vi "Get_MB_Setting.vi"(9 "DeviceName":string, 11 "DBRefNum":i32) -> (0 "Swap":T1, 1 "Mode":enum16{"RTU", "ASCII"}(ring), 2 "Address":string, 3 "DBRefNum Out":i32, 4 "Timeout":i32=1000, 5 "Device Index":u8, 6 "Name":string, 7 "Interval":u32)   [LabVIEW 2020, in "ModBus Serial Master.lvlib"]
uses:
  ModBus Serial Master.lvlib
  DriverCommon/Swap.ctl
  DriverCommon.lvlib
  SQLiteBase.lvlib
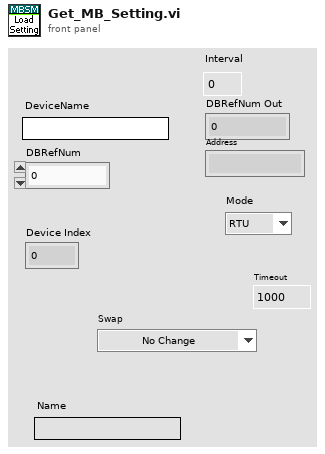
[diagram p1: front panel]
types:
  T1 = typedef "DriverCommon.lvlib/Swap.ctl" = enum16{"No Change", "Swap"}
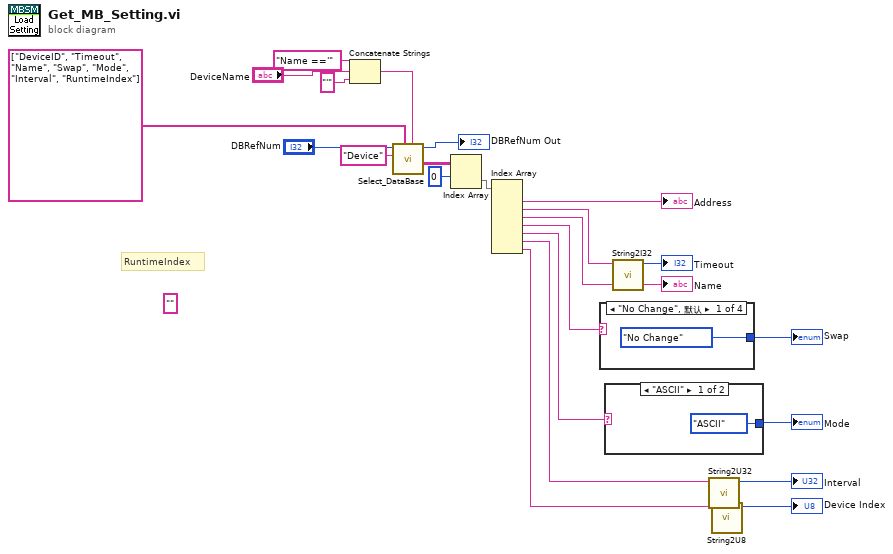
[diagram p0: block diagram]
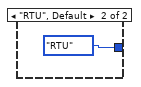
[diagram p2: hidden frame]
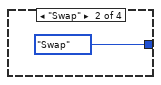
[diagram p3: hidden frame]
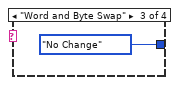
[diagram p4: hidden frame]
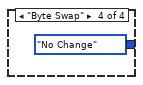
[diagram p5: hidden frame]
diagram:
  (unwired) "" ("Control Name")
  # "RuntimeIndex"
  n1 = Concatenate Strings("Name =='" ("Expression"), "DeviceName", "'" ("string")) -> (w18:string)
  n2 = call "Select_DataBase.vi"("Expression"=w18, "Query Columns"=string[] ["DeviceID", "Timeout", "Name", "Swap", "Mode", "Interval", "RuntimeIndex"], "Table name"="Device", "DB Reference In"="DBRefNum") -> ("Data"=w15:string[][], "DB Reference Out"=→"DBRefNum Out":i32)  [unwired: 5 in, 1 out]
  n3 = Index Array(array=w15, index (row)=0) -> (element=w13:string[])  [unwired: 1 in]
  n4 = Index Array(array=w13) -> (element #1=→"Address":string, element #2=w9:string, element #3=→"Name":string, element #4=w7:string, element #5=w5:string, element #6=w4:string, element #7=w2:string)  [unwired: 7 in]
  n5 = case shown="\"No Change\", 默认" w7 {
    tunnel: [Swap."No Change" ("Swap") Swap."Swap" ("Swap") Swap."No Change" ("Swap") Swap."No Change" ("Swap")] -> w10
    frame "No Change", Default {
    }
    frame "Swap" {
    }
    frame "Word and Byte Swap" {
    }
    frame "Byte Swap" {
    }
  }
  "Swap" <- w10
  n6 = case shown="\"ASCII\"" w5 {
    tunnel: [enum16{"RTU", "ASCII"}."ASCII" ("Mode") enum16{"RTU", "ASCII"}."RTU" ("Mode")] -> w6
    frame "ASCII" {
    }
    frame "RTU", Default {
    }
  }
  "Mode" <- w6
  n7 = call "String2I32.vi"("String"=w9) -> ("I32"=→"Timeout":i32)  [unwired: 10 in]
  n8 = call "String2U32.vi"("String"=w4) -> ("U32"=→"Interval":u32)  [unwired: 10 in]
  n9 = call "String2U8.vi"("String"=w2) -> ("U8"=→"Device Index":u8)  [unwired: 10 in]
